vi "Test Varint.vi"(8 "error in (no error)":errorcluster) -> (0 "error out":errorcluster)   [LabVIEW 2020]
uses:
  cdc024ba-9026-4d29-92d1-b4aac5bd19da.vi
  3c53edb6-61cf-4df4-a075-3edae7297449.vi
  d224062b-4249-40d3-b67c-8ad8b55e962a.vi
  89d6a59e-70c2-4d1d-ac08-29e0e6f3f6da.vi
  cdc024ba-9026-4d29-92d1-b4aac5bd19da.vi/45576c96-348a-4a29-82b0-147ecb2792d1.vi
  3c53edb6-61cf-4df4-a075-3edae7297449.vi/0f065a35-b637-42bd-ae45-04c3465bdb97.vi
  d224062b-4249-40d3-b67c-8ad8b55e962a.vi/e6afa5c7-117b-4965-af0c-e30c75561961.vi
  89d6a59e-70c2-4d1d-ac08-29e0e6f3f6da.vi/0f065a35-b637-42bd-ae45-04c3465bdb97.vi
  <vilib>/addons/_JKI Toolkits/Caraya/classes/Assert/Assert Equal Value_Variant.vi
  Source/Protobuf RAW.lvlib
  <vilib>/addons/_JKI Toolkits/Caraya/classes/Test/Test.lvclass
  <vilib>/addons/_JKI Toolkits/Caraya/classes/Assert/Assert.lvclass
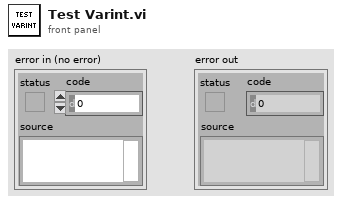
[diagram p1: front panel]
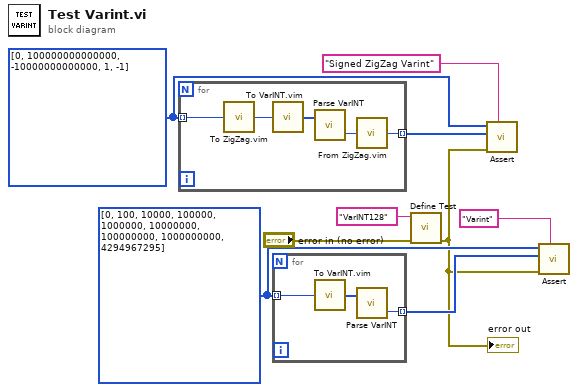
[diagram p0: block diagram]
diagram:
  w4 = i64[] [0, 100000000000000, -10000000000000, 1, -1] ("Signed Integer")
  w6 = u32[] [0, 100, 10000, 100000, 1000000, 10000000, 100000000, 1000000000, 4294967295]
  n1 = for {
    tunnel: w4 -> [w11] mode=indexing
    tunnel: [w10] -> w5 mode=indexing
    n2 = call "To ZigZag.vim"("Signed Integer"=w11) -> ("Zig Zag"=w13:u64)
    n3 = call "To VarINT.vim"("Integer"=w13) -> ("LEB128"=w14:u8[])
    n4 = call "Parse VarINT.vi"("Buffer"=w14) -> ("Numeric"=w12:u64)  [unwired: 1 in, 1 out]
    n5 = call "From ZigZag.vim"("ZigZag"=w12) -> ("Signed Integer"=w10:i64)
  }
  n6 = for {
    tunnel: [w16] -> w8 mode=indexing
    tunnel: w6 -> [w15] mode=indexing
    n7 = call "To VarINT.vim"("Integer"=w15) -> ("LEB128"=w17:u8[])
    n8 = call "Parse VarINT.vi"("Buffer"=w17) -> ("Numeric"=w16:u64)  [unwired: 1 in, 1 out]
  }
  n9 = call <vilib>:"Define Test.vi"("error in (no error)"="error in (no error)", "Label (VI Title)"="VarINT128") -> ("error out"=w2:errorcluster)  [unwired: 9 in]
  "error out" <- w2
  n10 = call-poly <vilib>:"Assert.vi"("Label"="Signed ZigZag Varint", "error in (no error)"=w2, "Y"=w5, "X"=w4) -> ()  [unwired: 7 in, 1 out]
  n11 = call-poly <vilib>:"Assert.vi"("Label"="Varint", "error in (no error)"=w2, "Y"=w8, "X"=w6) -> ()  [unwired: 7 in, 1 out]
